vi "sub_main_udp.vi"(8 "error in":errorcluster) -> (0 "error out":errorcluster)   [LabVIEW 2019]
panel:
  out "결과 문자열":string
  out "data out":string
  out "문자열 2":string
  in  "문자열":string
  out "loop":i32
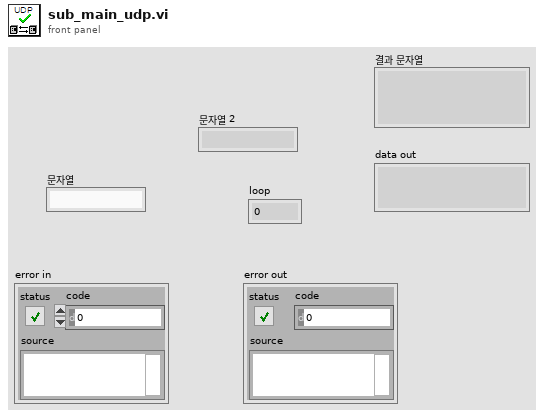
[diagram p1: front panel]
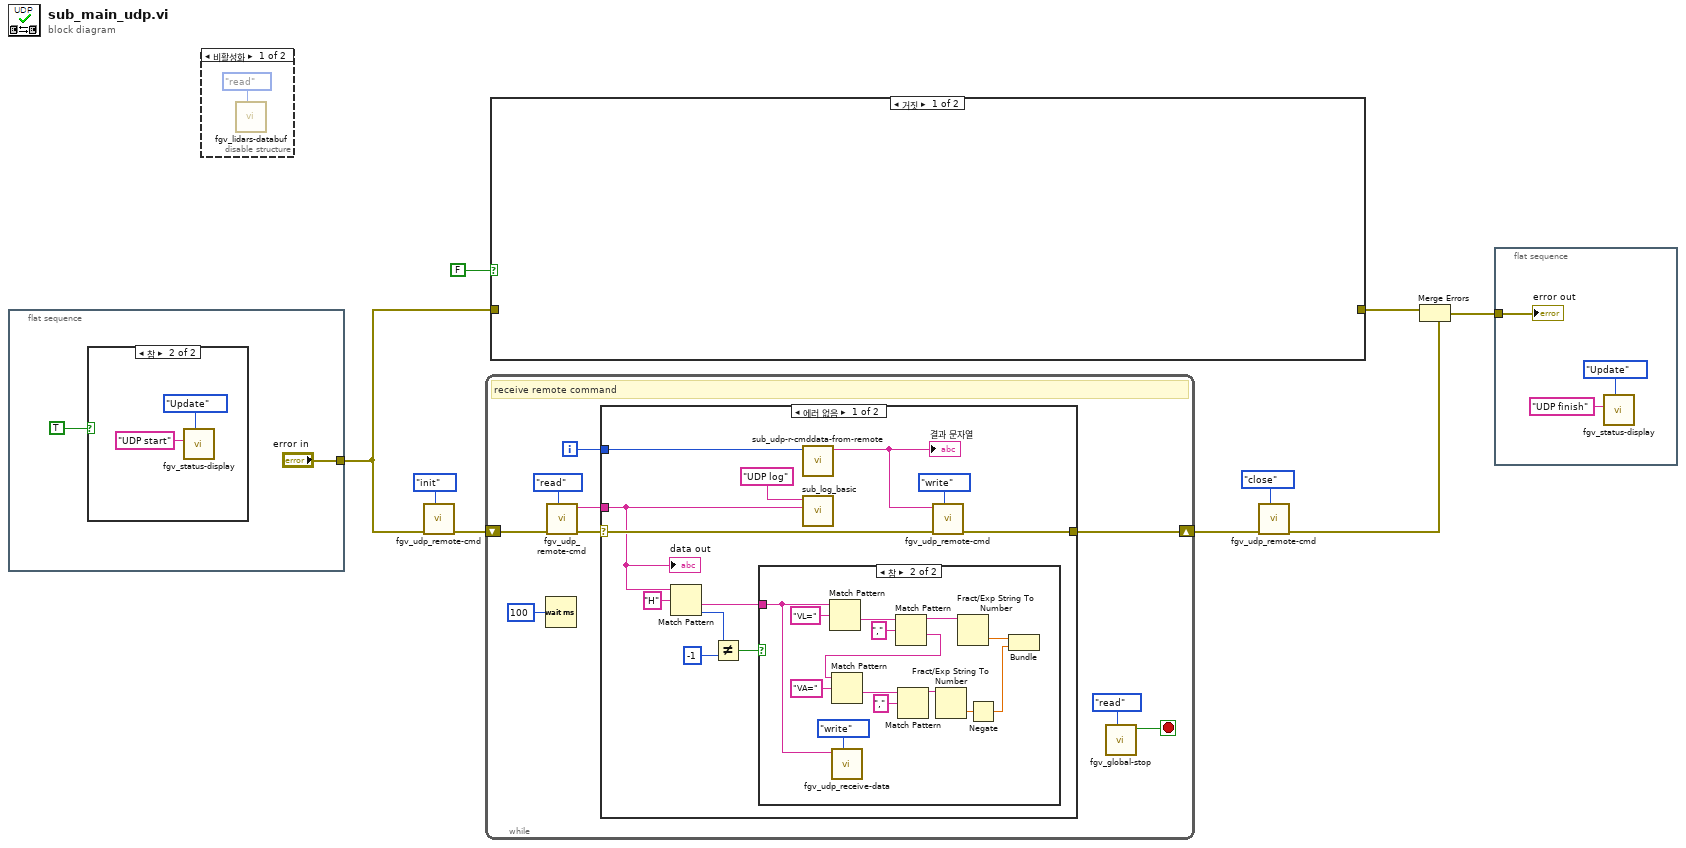
[diagram p0: block diagram]
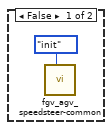
[diagram p2: hidden frame]
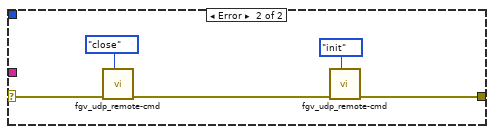
[diagram p3: hidden frame]
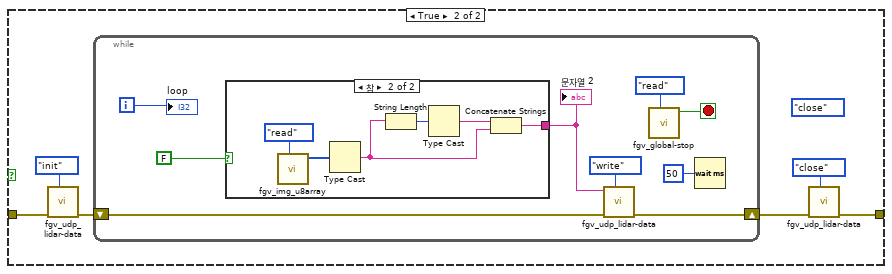
[diagram p4: hidden frame]
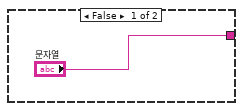
[diagram p5: hidden frame]
diagram:
  n1 = flat-sequence {
    tunnel: ["error in"] -> w9
    frame #0 {
      n2 = case shown="참" TRUE {
        frame False {
        }
        frame True {
          n3 = call "fgv_status-display.vi"("Mode"=enum16{"Initial", "Update", "Clear"}."Update", "title"="UDP start" ("String in 1")) -> ()  [unwired: 9 in, 1 out]
        }
      }
    }
  }
  n4 = disable-structure shown="비활성화" {
    frame Disabled {
      n5 = call "fgv_lidars-databuf.vi"("cmd"=enum16{"ini img arr", "write", "read"}."read") -> ()  [unwired: 9 in, 2 out]
    }
    frame Enabled {
    }
  }
  n6 = call "fgv_udp_remote-cmd.vi"("cmd"=enum16{"init", "read", "write", "close"}."init", "error in"=w9) -> ("error out"=w4:errorcluster)  [unwired: 8 in, 1 out]
  n7 = while {
    shift-right: [w17] -> w3
    shift-left: w4 -> [w22]
    i -> [w15]
    stop <- w19 stop-if-true
    # "receive remote command"
    n8 = Wait (ms)(milliseconds to wait=u32 100) -> ()  [unwired: 1 out]
    n9 = call "fgv_udp_remote-cmd.vi"("cmd"=enum16{"init", "read", "write", "close"}."read", "error in"=w22) -> ("error out"=w18:errorcluster, "data out"=w16:string)  [unwired: 8 in]
    n10 = case shown="에러 없음" w18 {
      selector: w18 -> [w27 w53]
      tunnel: [w29 w51] -> w17
      tunnel: w16 -> [w26 _]
      tunnel: w15 -> [w24 _]
      frame No Error {
        n11 = Match Pattern(string=w26, regular expression="H" ("정규식")) -> (after substring=w31:string, offset past match=w34:i32)  [unwired: 1 in, 2 out]
        n12 = Not Equal?(x=w34, y=-1) -> (x != y?=w32:bool)
        n13 = case shown="참" w32 {
          tunnel: w31 -> [_ w38]
          frame False {
            n14 = call "fgv_agv_speedsteer-common.vi"("cmd"=enum16{"init", "read", "write"}."init") -> ()  [unwired: 9 in, 2 out]
          }
          frame True {
            n15 = Match Pattern(string=w38, regular expression="VL=" ("정규식")) -> (after substring=w48:string)  [unwired: 1 in, 3 out]
            n16 = call "fgv_udp_receive-data.vi"("cmd"=enum16{"read", "write"}."write", "receive buff"=w38) -> ()  [unwired: 9 in, 1 out]
            n17 = Match Pattern(string=w48, regular expression="," ("정규식")) -> (before substring=w47:string, after substring=w42:string)  [unwired: 1 in, 2 out]
            n18 = Match Pattern(string=w42, regular expression="VA=" ("정규식")) -> (after substring=w45:string)  [unwired: 1 in, 3 out]
            n19 = Match Pattern(string=w45, regular expression="," ("정규식")) -> (before substring=w46:string)  [unwired: 1 in, 3 out]
            n20 = Fract/Exp String To Number(string=w46) -> (number=w41:dbl)  [unwired: 3 in, 1 out]
            n21 = Fract/Exp String To Number(string=w47) -> (number=w40:dbl)  [unwired: 3 in, 1 out]
            n22 = Negate(x=w41) -> (-x=w39:dbl)
            n23 = Bundle(w40, w39) -> ()  [unwired: 1 in, 1 out]
          }
        }
        n24 = call "sub_udp-r-cmddata-from-remote.vi"("index"=w24) -> ("udp send data"=w25:string)  [unwired: 10 in]
        "결과 문자열" <- w25
        n25 = call "sub_log_basic.vi"("desc"=w26, "Title"="UDP log") -> ()  [unwired: 9 in, 1 out]
        n26 = call "fgv_udp_remote-cmd.vi"("cmd"=enum16{"init", "read", "write", "close"}."write", "error in"=w27, "data in"=w25) -> ("error out"=w29:errorcluster)  [unwired: 7 in, 1 out]
        "data out" <- w26
      }
      frame Error {
        n27 = call "fgv_udp_remote-cmd.vi"("cmd"=enum16{"init", "read", "write", "close"}."close", "error in"=w53) -> ("error out"=w52:errorcluster)  [unwired: 8 in, 1 out]
        n28 = call "fgv_udp_remote-cmd.vi"("cmd"=enum16{"init", "read", "write", "close"}."init", "error in"=w52) -> ("error out"=w51:errorcluster)  [unwired: 8 in, 1 out]
      }
    }
    n29 = call "fgv_global-stop.vi"("cmd"=enum16{"init", "stop", "read"}."read") -> ("val_out"=w19:bool)  [unwired: 10 in]
  }
  n30 = case shown="거짓" FALSE {
    tunnel: w9 -> [_ w61]
    tunnel: [_ w58] -> w7
    frame False {
    }
    frame True {
      (unwired) enum16{"init", "read", "write", "close"}."close" ("cmd")
      n31 = call "fgv_udp_lidar-data.vi"("cmd"=enum16{"init", "r-w", "read", "write", "close"}."init", "error in"=w61) -> ("error out"=w60:errorcluster)  [unwired: 7 in, 2 out]
      n32 = while {
        shift-right: [w68] -> w59
        shift-left: w60 -> [w69]
        i -> [w63]
        stop <- w66 stop-if-true
        n33 = case shown="참" FALSE ("불리언") {
          tunnel: ["문자열" w72] -> w65
          frame False {
          }
          frame True {
            n34 = call "fgv_img_u8array.vi"("cmd"=enum16{"init", "read", "write"}."read") -> ("image array"=w75:u8[])  [unwired: 10 in]
            n35 = Type Cast(x=w75) -> (*(type *) &x=w73:string)  [unwired: 1 out]
            n36 = String Length(string=w73) -> (length=w76:i32)
            n37 = Type Cast(x=w76) -> (*(type *) &x=w74:string)  [unwired: 1 out]
            n38 = Concatenate Strings(w74, w73) -> (w72:string)
          }
        }
        "문자열 2" <- w65
        n39 = call "fgv_udp_lidar-data.vi"("cmd"=enum16{"init", "r-w", "read", "write", "close"}."write", "error in"=w69, "data in"=w65) -> ("error out"=w68:errorcluster)  [unwired: 6 in, 2 out]
        n40 = call "fgv_global-stop.vi"("cmd"=enum16{"init", "stop", "read"}."read") -> ("val_out"=w66:bool)  [unwired: 10 in]
        n41 = Wait (ms)(milliseconds to wait=u32 50) -> ()  [unwired: 1 out]
        "loop" <- w63
      }
      n42 = call "fgv_udp_lidar-data.vi"("cmd"=enum16{"init", "r-w", "read", "write", "close"}."close", "error in"=w59) -> ("error out"=w58:errorcluster)  [unwired: 7 in, 2 out]
    }
  }
  n43 = call "fgv_udp_remote-cmd.vi"("cmd"=enum16{"init", "read", "write", "close"}."close", "error in"=w3) -> ("error out"=w8:errorcluster)  [unwired: 8 in, 1 out]
  n44 = Merge Errors(w7, w8) -> (w6:errorcluster)
  n45 = flat-sequence {
    tunnel: w6 -> [w78]
    frame #0 {
      n46 = call "fgv_status-display.vi"("Mode"=enum16{"Initial", "Update", "Clear"}."Update", "title"="UDP finish" ("String in 1")) -> ()  [unwired: 9 in, 1 out]
      "error out" <- w78
    }
  }
